vi "RCV Test.vi"(0 "Semiconductor Module Context":T5, 2 "Test Information":T6={"Exp Name"="Cold Switching", "Lot"="0233A", "Wafer"="15", "Die Type"="L22", "Die X "="6", "Die Y"="8", "Exp"="1", "Die X_Y"="8"}, 5 "Sweep Settings":T3={"Start"=0.0, "Stop"=1.0, "Step"=0.0}, 7 "Test_Pins":T2={"RF_Pins"=["RF1", "RF2"], "Contact_Meas_Pins"=["RF1"], "Contact_Source_Pins"=["RF1"], "Sweep_Bias_Pins"=[]}, 9 "error in (no error)":errorcluster) -> (6 "Meaurements":T1, 13 "S11":string[](array[string]), 14 "S22":string[](array[string]), 15 "error out":errorcluster)   [LabVIEW 2013]
doc: "Initiates and fetches niVNA S11 measurements and converts it to a capacitance measurement."
uses:
  <vilib>/NI_TestStand_SemiconductorModule/NI_TestStand_Semiconductor_Module.lvlibp/PinMap/General/SemiconductorModuleContext.ctl
  Controls/Sweep Settings.ctl
  Controls/Test_Pins.ctl
  Controls/Measurements.ctl
  Controls/Test Information.ctl
  <vilib>/NI_TestStand_SemiconductorModule/NI_TestStand_Semiconductor_Module.lvlibp
panel:
  out "Graph Cluster":T4
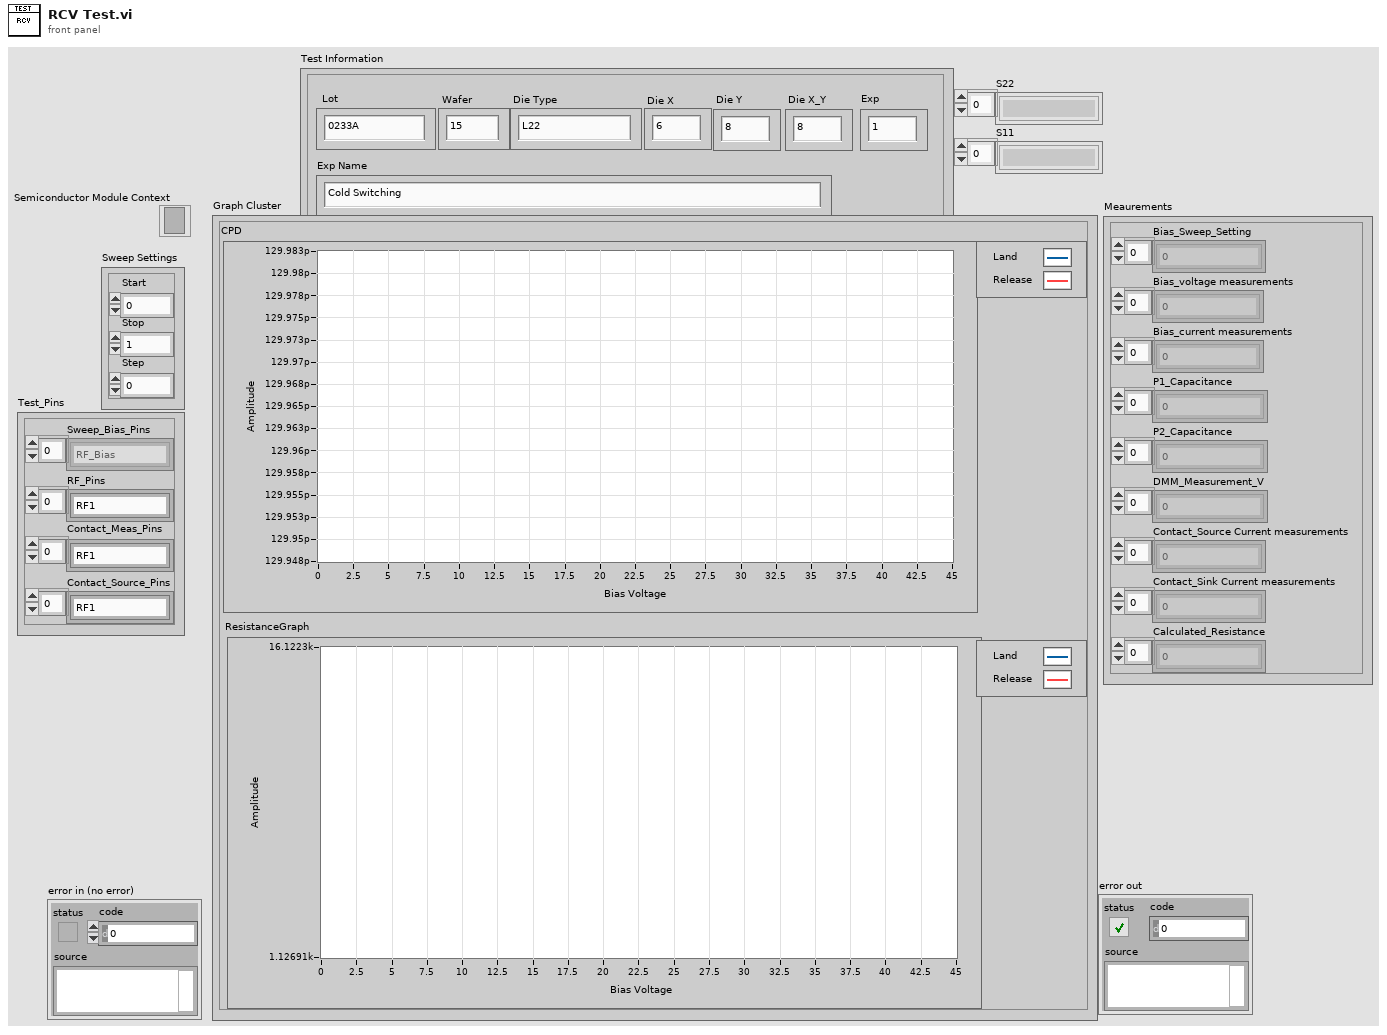
[diagram p1: front panel]
types:
  T1 = typedef "Measurements.ctl" = cluster{"Bias_voltage measurements":dbl[], "Bias_current measurements":dbl[], "P1_Capacitance":dbl[], "P2_Capacitance":dbl[], "DMM_Measurement_V":dbl[], "Bias_Sweep_Setting":dbl[], "Contact_Source Current measurements":dbl[], "Contact_Sink Current measurements":dbl[], "Calculated_Resistance":dbl[]}
  T2 = typedef "Test_Pins.ctl" = cluster{"RF_Pins":string[], "Contact_Meas_Pins":string[], "Contact_Source_Pins":string[], "Sweep_Bias_Pins":string[]}
  T3 = typedef "Sweep Settings.ctl" = cluster{"Start":dbl, "Stop":dbl, "Step":dbl}
  T4 = cluster{"ResistanceGraph":cluster{dbl[], dbl[]}[], "CPD":cluster{dbl[], dbl[]}[]}
  T5 = typedef "NI_TestStand_Semiconductor_Module.lvlibp/SemiconductorModuleContext.ctl" = refnum<k7>
  T6 = typedef "Test Information.ctl" = cluster{"Exp Name":string, "Lot":string, "Wafer":string, "Die Type":string, "Die X ":string, "Die Y":string, "Exp":string, "Die X_Y":string}
  T7 = typedef "imagedata.ctl" = cluster{"image type":i32, "image depth":i32, "image":u8[], "mask":u8[], "colors":u32[], "Rectangle":cluster{"left":i16, "top":i16, "right":i16, "bottom":i16}}
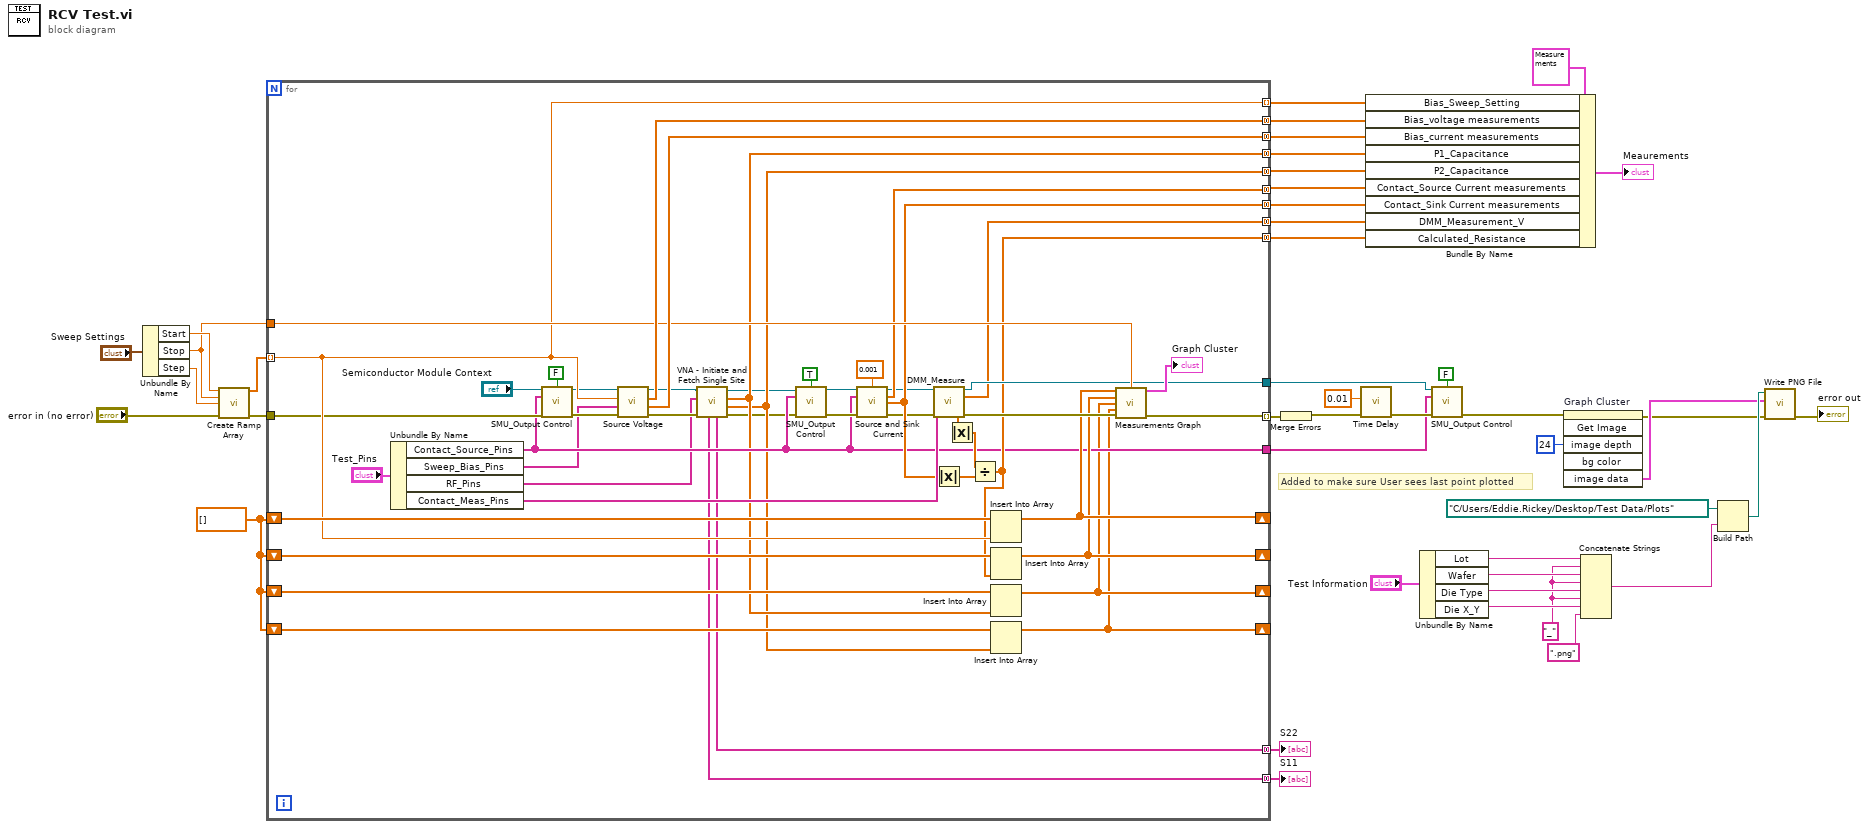
[diagram p0: block diagram]
diagram:
  w11 = "_"
  w35 = dbl[] []
  # "Added to make sure User sees last point plotted"
  n1 = Unbundle By Name("Sweep Settings") -> ("Start"=w38:dbl, "Stop"=w36:dbl, "Step"=w37:dbl)
  n2 = call "Create Ramp Array.vi"("Start"=w38, "Stop"=w36, "Step"=w37, "Error In"="error in (no error)") -> ("Ramp Pattern"=w43:dbl[], "Error Out"=w40:errorcluster)  [unwired: 10 in]
  n3 = for {
    tunnel: w43 -> [w75] mode=indexing
    tunnel: [w89] -> w25 mode=concatenating
    tunnel: [w88] -> w24 mode=concatenating
    tunnel: [w53] -> w23 mode=concatenating
    tunnel: [w52] -> w22 mode=concatenating
    tunnel: [w61] -> w19 mode=concatenating
    tunnel: [w86] -> w42 mode=indexing
    tunnel: w40 -> [w74]
    tunnel: w36 -> [w82]
    shift-right: [w81] -> _
    shift-left: w35 -> [w80]
    shift-right: [w79] -> _
    shift-left: w35 -> [w78]
    shift-right: [w55] -> _
    shift-left: w35 -> [w77]
    shift-right: [w54] -> _
    shift-left: w35 -> [w76]
    tunnel: [w75] -> w26 mode=indexing
    tunnel: [w67] -> w30
    tunnel: [w56] -> w29
    tunnel: [w66] -> w21 mode=concatenating
    tunnel: [w64] -> w20 mode=concatenating
    tunnel: [w63] -> w18 mode=concatenating
    tunnel: [w45] -> w1 mode=concatenating
    tunnel: [w44] -> w2 mode=concatenating
    n4 = Unbundle By Name("Test_Pins") -> ("Contact_Source_Pins"=w56:string[], "Sweep_Bias_Pins"=w46:string[], "RF_Pins"=w47:string[], "Contact_Meas_Pins"=w83:string[])
    n5 = call "SMU_Output Control.vi"("Semiconductor Module Context"="Semiconductor Module Context", "output enabled?"=FALSE, "Pins"=w56, "error in (no error)"=w74) -> ("Semiconductor Module Context Out"=w71:T5, "error out"=w73:errorcluster)  [unwired: 10 in]
    n6 = call "Source Voltage.vi"("error in (no error)"=w73, "Pins"=w46, "voltage level"=w75, "Semiconductor Module Context"=w71) -> ("error out"=w51:errorcluster, "current measurements"=w88:dbl[], "voltage measurements"=w89:dbl[], "Semiconductor Module Context Out"=w49:T5)  [unwired: 4 in]
    n7 = call "VNA - Initiate and Fetch Single Site.vi"("error in (no error)"=w51, "Pins"=w47, "Semiconductor Module Context"=w49) -> ("error out"=w50:errorcluster, "P2_Capacitance"=w52:dbl[], "P1_Capacitance"=w53:dbl[], "Semiconductor Module Context Out"=w48:T5, "S22"=w44:string[], "S11"=w45:string[])  [unwired: 3 in]
    n8 = call "SMU_Output Control.vi"("Semiconductor Module Context"=w48, "output enabled?"=TRUE, "Pins"=w56, "error in (no error)"=w50) -> ("Semiconductor Module Context Out"=w57:T5, "error out"=w58:errorcluster)  [unwired: 10 in]
    n9 = call "Source and Sink Current.vi"("Semiconductor Module Context"=w57, "Current level"=0.001, "Pins"=w56, "error in (no error)"=w58) -> ("Semiconductor Module Context Out"=w59:T5, "Source Current measurements"=w66:dbl[], "Sink Current measurements"=w64:dbl[], "error out"=w60:errorcluster)  [unwired: 8 in]
    n10 = call "DMM_Measure.vi"("Semiconductor Module Context"=w59, "Pins"=w83, "Error In"=w60) -> ("Semiconductor Module Context Out"=w67:T5, "Measurement"=w61:dbl[], "Error Out"=w87:errorcluster)  [unwired: 10 in]
    n11 = Absolute Value(x=w64) -> (abs(x)=w65:dbl[])
    n12 = Absolute Value(x=w61) -> (abs(x)=w62:dbl[])
    n13 = Divide(x=w62, y=w65) -> (x/y=w63:dbl[])
    n14 = Insert Into Array(array=w80, new element=w75) -> (w81:dbl[])  [unwired: 1 in]
    n15 = Insert Into Array(array=w78, new element=w63) -> (w79:dbl[])  [unwired: 1 in]
    n16 = Insert Into Array(array=w77, new element=w53) -> (w55:dbl[])  [unwired: 1 in]
    n17 = Insert Into Array(array=w76, new element=w52) -> (w54:dbl[])  [unwired: 1 in]
    n18 = call "Measurements Graph.vi"("Bias Voltage"=w81, "Stop_V"=w82, "Resitance"=w79, "Port 1 Cap"=w55, "Port 2 Cap"=w54, "Error In"=w87) -> ("Graph Cluster"=→"Graph Cluster":T4, "Error Out"=w86:errorcluster)  [unwired: 8 in]
  }
  "S22" <- w2
  "S11" <- w1
  n19 = Merge Errors(w42) -> (w33:errorcluster)
  n20 = call "Time Delay"("error in (no error)"=w33, "Delay Time (s)"=0.01) -> ("error out"=w31:errorcluster)  [unwired: 9 in]
  n21 = Bundle By Name(cluster=T1 {"Bias_voltage measurements"=[4.932090623749482e-05, 1.0000316998790688, 2.000000012027978, 3.0000105246486535, 4.000063237741095, 5.000059683537849, 5.999999862038914, 6.999996307835667, 7.999992753632419, 9.00003139990094, 9.999971578402006, 11.000010224670525, 12.000006670467277, 13.00000311626403, 14.000013628884707, 15.000024141505381, 15.999964320006447, 16.999988899451044, 18.000013478895642, 18.99998179104455, 19.999992303665227, 21.000016883109826, 22.000041462554424, 22.999953507407643, 24.000034354147928, 24.999890131705463, 26.0000694462132, 27.000009624714263, 28.000006070511017, 28.999974382659925, 29.999928627984918, 31.000009474725204, 32.00006218781765, 33.00004456679048, 33.99995661164369, 34.99996712426437, 36.00006203782858, 37.00005848362534, 37.99998459530247, 39.00000917474708, 39.99993528642421, 39.999977486895986, 38.9999669742753, 37.99998459530247, 36.99998814950572, 36.000047971004655, 35.00003745838398, 34.000041012587225, 32.99996016584694, 32.00000592052195, 31.000037608373045, 29.999998962104527, 29.00004471677954, 28.000034204158865, 26.999995557890347, 26.0000694462132, 24.99994639900115, 23.999964020028315, 22.999995707879407, 21.999999262082657, 20.99998874946198, 20.000034504136995, 18.99996772422063, 18.000027545719565, 17.000045166746734, 16.000020587302135, 14.999981941033615, 13.999999562060784, 12.999960915792265, 12.000048870939043, 10.999953957374835, 9.999971578402006, 9.000003266253096, 7.999964619984577, 6.999968174187822, 5.999985795214991, 4.999989349418239, 3.9999929036214845, 2.999982391000809, 1.999971878380134, 1.0000176330551467, -6.946389450834399e-06], "Bias_current measurements"=[-1.3036076216311926e-06, -1.2473205913364035e-06, -1.275464106483798e-06, -1.1066030155988914e-06, -1.2191770761888292e-06, -1.3036076216311926e-06, -1.331751136778767e-06, -1.1628900458938604e-06, -1.275464106483798e-06, -1.2191770761888292e-06, -1.1628900458938604e-06, -1.3036076216311926e-06, -1.3036076216311926e-06, -1.1066030155988914e-06, -1.134746530746466e-06, -1.3036076216311926e-06, -1.191033561041435e-06, -1.134746530746466e-06, -1.3036076216311926e-06, -1.191033561041435e-06, -1.1628900458938604e-06, -9.658854398615593e-07, -1.0503159853039228e-06, -1.2191770761888292e-06, -1.0503159853039228e-06, -1.1066030155988914e-06, -1.191033561041435e-06, -1.0221724701565283e-06, -1.191033561041435e-06, -1.191033561041435e-06, -1.0221724701565283e-06, -1.1628900458938604e-06, -1.0784595004514971e-06, -1.3598946519261614e-06, -1.1628900458938604e-06, -1.191033561041435e-06, -1.0221724701565283e-06, -1.0784595004514971e-06, -1.0221724701565283e-06, -1.1628900458938604e-06, -1.1066030155988914e-06, -1.4724687125160992e-06, -1.4443251973687047e-06, -1.3036076216311926e-06, -1.3036076216311926e-06, -1.331751136778767e-06, -1.3598946519261614e-06, -1.5006122276636737e-06, -1.5850427731060368e-06, -1.5850427731060368e-06, -1.5568992579586423e-06, -1.4443251973687047e-06, -1.3598946519261614e-06, -1.4724687125160992e-06, -1.4161816822211302e-06, -1.4724687125160992e-06, -1.5006122276636737e-06, -1.6131862882536113e-06, -1.4161816822211302e-06, -1.528755742811068e-06, -1.5568992579586423e-06, -1.5568992579586423e-06, -1.4724687125160992e-06, -1.5568992579586423e-06, -1.4161816822211302e-06, -1.3880381670737359e-06, -1.331751136778767e-06, -1.5006122276636737e-06, -1.6413298034010058e-06, -1.4443251973687047e-06, -1.5850427731060368e-06, -1.5568992579586423e-06, -1.5006122276636737e-06, -1.6131862882536113e-06, -1.6976168336959744e-06, -1.6413298034010058e-06, -1.4161816822211302e-06, -1.5850427731060368e-06, -1.528755742811068e-06, -1.5006122276636737e-06, -1.4443251973687047e-06, -1.528755742811068e-06], "P1_Capacitance"=[1.445308224781364e-14, 1.3825341111416653e-14, 1.6610608612578052e-14, 1.5895159215281275e-14, 1.4601425796382007e-14, 1.6320337037148908e-14, 1.6656100654703588e-14, 1.3010650904799276e-14, 1.2332669244279774e-14, 1.2821431569149479e-14, 1.3112696687725679e-14, 1.293724489255816e-14, 1.2556760931602158e-14, 1.253968061657498e-14, 1.2784161027418273e-14, 1.585925318437538e-14, 1.2800225565312751e-14, 1.2666746777283852e-14, 1.500714808802598e-14, 1.195485242522037e-14, 1.448487961996781e-14, 1.4822860098338094e-14, 1.3862431633706082e-14, 1.2961374453184943e-14, 1.1806930259008016e-14, 7.076389460329639e-15, 5.99546323151383e-15, 1.0748007126477565e-14, 1.0013590697177481e-14, 5.410646172186829e-15, 1.0247044254101682e-14, 3.827760979246635e-15, 5.867028076477222e-15, 5.257170136006713e-15, 6.5302151222389694e-15, 7.000448041298376e-15, 7.749625187630852e-15, 8.485636759835786e-15, 1.0581626944240925e-14, 9.429825860775007e-15, 8.111448046349839e-15, 8.08954332506056e-15, 1.1955330233344829e-14, 1.2464897359343811e-14, 1.3331085376088181e-14, 6.888420149302219e-15, 1.3841889105112939e-14, 1.4015385900382396e-14, 5.644362604048724e-15, 6.1655681308297405e-15, 7.27033745575812e-15, 7.759236524135619e-15, 9.2501949188729e-15, 1.2724642521178732e-14, 9.66398512641692e-15, 1.1179237950851952e-14, 1.0856173907305758e-14, 1.1142614117732694e-14, 1.0416396084636245e-14, 1.1581741072610669e-14, 1.0880136394130115e-14, 1.1841005835382791e-14, 1.2817811881176867e-14, 1.2493927775974342e-14, 1.074359787812355e-14, 9.934245844842753e-15, 1.341076243695591e-14, 1.3328375502821986e-14, 1.1232341726300313e-14, 1.3970994202658144e-14, 1.2678537188068271e-14, 1.4707972558159856e-14, 1.3405016690896814e-14, 1.428112271375313e-14, 1.320134178171383e-14, 1.431000600900096e-14, 1.3491400002556214e-14, 1.4335881913082714e-14, 1.3972909633251083e-14, 1.5835755092405272e-14, 1.5117696585258153e-14, 1.7141448347318333e-14], "P2_Capacitance"=[9.98769428790146e-15, 9.589982366669586e-15, 9.641938536867875e-15, 9.501362686341329e-15, 1.0334120913933413e-14, 8.335359508073015e-15, 9.76050509259481e-15, 9.768224818585788e-15, 8.667636761358e-15, 8.539875122144578e-15, 7.523853186493658e-15, 7.44619299711258e-15, 8.693993993274902e-15, 5.7007159893247856e-15, 8.112011488523546e-15, 6.41842965312186e-15, 2.7560404916430395e-15, 1.6146654420062674e-15, 9.18712261738975e-16, 2.8499977600410103e-15, 4.309012006954116e-16, 2.4884754788857034e-15, -5.150733166780367e-16, 1.8043683251639506e-15, 1.878051630521273e-15, 1.109231805531228e-15, 2.9722275010185344e-15, 4.69727992114551e-16, 3.2570208474803507e-15, 3.377721019381114e-15, 7.112810669699152e-16, 5.252794248525848e-15, 4.3635239030802064e-15, 2.6702944555657184e-15, 5.082049013134563e-15, 3.9171585852766245e-15, 1.7918951967318813e-15, 3.5079109322806944e-15, 2.253293636724557e-15, 1.9417257460719145e-15, -4.3985350924570067e-16, -1.5442724892074044e-16, 1.217951694733645e-15, 1.3829209803368947e-15, 8.962076623113751e-16, 2.0945517931301525e-15, -3.4146986700553743e-16, 2.560447163009517e-15, -5.81016832931674e-16, 3.50356867358908e-15, 3.1033234645204277e-15, 2.830602805149267e-15, 3.189862103276134e-15, 4.8762072259606355e-15, 4.425199586558695e-15, 3.770331130106188e-15, 4.573601303416273e-15, 1.061820842248423e-14, 4.526023808494307e-15, 1.3375064579710585e-14, 1.3303940031568891e-14, 1.3655393097065122e-14, 2.691700139513934e-15, 2.9679270948978025e-15, 1.4758562028593512e-14, 2.7917747354728885e-15, 1.4004725917895709e-14, 1.4480595113010032e-14, 1.3012823302883627e-14, 1.2567189118302562e-14, 1.243616195763473e-14, 9.254690061898573e-15, 7.878495056502322e-15, 1.0999170120610966e-14, 1.3230685711209752e-14, 1.1232722152618156e-14, 1.3399651102686109e-14, 1.2603050688562835e-14, 1.3383365659395111e-14, 1.4777927887074333e-14, 1.483326519845907e-14, 1.4275658415133204e-14], "DMM_Measurement_V"=[0.00010147032237547078, 9.081499934906936e-05, 9.455424649421084e-05, 0.000118362364393024, 8.180795205604426e-05, 0.00010272880317189954, 0.00010941100209099095, 9.720206781590102e-05, 9.238531609505587e-05, 8.666646752013347e-05, 9.68039201303053e-05, 0.00010813581579726455, 9.957703268172797e-05, 0.00010424621917644314, 0.00010365038977282434, 0.00010332184832596885, 8.947299106615186e-05, 8.659129278229347e-05, 0.00011768022325336672, 0.00011335071520370539, 9.742759202942038e-05, 7.846685259649825e-05, 0.00010495898706114637, 0.00012124963117598138, 8.280192914525899e-05, 0.00010158447660700506, 0.00011284119753612472, 0.00011378227388389648, 9.934593996910943e-05, 0.00010268703942865523, 7.153685546749087e-05, 9.692921136003808e-05, 0.0001139966610992175, 6.041377851675279e-05, 0.00011679483189658697, 9.262476155632308e-05, 0.00010875113494773059, 0.0001028485259025332, 0.00011064720889102295, 7.809654740639858e-05, 6.909785286202215e-05, 0.00011470942898392074, 7.079346083774157e-05, 0.0001100541637369535, 0.00010617291986478143, 0.00010530144975574979, 8.210308250830383e-05, 6.7390156991509816e-06, 3.865670163941557e-06, -7.088518460863526e-07, 1.4962737972136345e-06, 4.416951574766798e-06, 1.8053254972219903e-06, 6.240635029768443e-06, -2.4388217129950166e-07, 1.3765510665799904e-06, 3.876807162139957e-06, -3.998001460785389e-07, 2.4345658954363024e-06, 9.422081368390276e-07, 1.1649481008089936e-06, 3.4424642323991434e-06, 2.4429186440850517e-06, -8.397115749183832e-07, 3.6345774513230587e-06, 5.9761313225544595e-06, 1.99187021704636e-06, 2.8438505792305975e-06, -3.5153753921046856e-06, 6.240635029768727e-06, -3.6545878695860075e-06, 1.783728636483065e-08, 1.4034426654803075e-07, 4.68145528198074e-06, 5.802556953883901e-07, 2.5069563837263568e-06, 4.9403904900954625e-06, 8.029956593578547e-07, 7.045283149609185e-06, 1.2651810845951768e-06, -1.4522464758351698e-06, 4.3195028405297234e-06], "Bias_Sweep_Setting"=[0.0, 1.0, 2.0, 3.0, 4.0, 5.0, 6.0, 7.0, 8.0, 9.0, 10.0, 11.0, 12.0, 13.0, 14.0, 15.0, 16.0, 17.0, 18.0, 19.0, 20.0, 21.0, 22.0, 23.0, 24.0, 25.0, 26.0, 27.0, 28.0, 29.0, 30.0, 31.0, 32.0, 33.0, 34.0, 35.0, 36.0, 37.0, 38.0, 39.0, 40.0, 40.0, 39.0, 38.0, 37.0, 36.0, 35.0, 34.0, 33.0, 32.0, 31.0, 30.0, 29.0, 28.0, 27.0, 26.0, 25.0, 24.0, 23.0, 22.0, 21.0, 20.0, 19.0, 18.0, 17.0, 16.0, 15.0, 14.0, 13.0, 12.0, 11.0, 10.0, 9.0, 8.0, 7.0, 6.0, 5.0, 4.0, 3.0, 2.0, 1.0, 0.0], "Contact_Source Current measurements"=[], "Contact_Sink Current measurements"=[], "Calculated_Resistance"=[]} ("Meaurements 2"), "Bias_Sweep_Setting"=w26, "Bias_voltage measurements"=w25, "Bias_current measurements"=w24, "P1_Capacitance"=w23, "P2_Capacitance"=w22, "Contact_Source Current measurements"=w21, "Contact_Sink Current measurements"=w20, "DMM_Measurement_V"=w19, "Calculated_Resistance"=w18) -> (→"Meaurements":T1)
  n22 = Unbundle By Name("Test Information") -> ("Lot"=w15:string, "Wafer"=w14:string, "Die Type"=w13:string, "Die X_Y"=w12:string)
  n23 = call "SMU_Output Control.vi"("Semiconductor Module Context"=w30, "output enabled?"=FALSE, "Pins"=w29, "error in (no error)"=w31) -> ("error out"=w17:errorcluster)  [unwired: 10 in, 1 out]
  n24 = invoke on="Graph Cluster" class="Clust (strict)" method="Get Image"(error in=w17, "image depth"=24 ("Image Depth")) -> (error out=w3:errorcluster, "image data"=w5:T7)  [unwired: 4 in, 4 out]
  n25 = Concatenate Strings(w15, w11, w14, w11, w13, w11, w12, ".png" ("string")) -> (w10:string)
  n26 = Build Path(base path=path "C:/Users/Eddie.Rickey/Desktop/Test Data/Plots", name or relative path=w10) -> (appended path=w6:path)
  n27 = call <vilib>:"Write PNG File.vi"("error in (no error)"=w3, "image data"=w5, "path to PNG file"=w6) -> ("error out"=→"error out":errorcluster)  [unwired: 7 in, 1 out]
